vi "RemovePMUModule.vi"(8 "Error In":errorcluster[](array[cluster]), 11 "Bus in":refnum<class "Bus.lvclass">) -> (0 "Error Out":errorcluster[](array[cluster]), 3 "Bus out":refnum<class "Bus.lvclass">)   [LabVIEW 2014]
uses:
  Bus.lvclass
  <userlib>/NIST/NistModuleAdminLib/NistModuleAdmin/NistModuleAdmin.lvclass
  <userlib>/NIST/NISTErrorLib/NISTErrorLib.lvlib
  PmuImpairment/PmuImpairModule/PmuImpairModule.lvlib
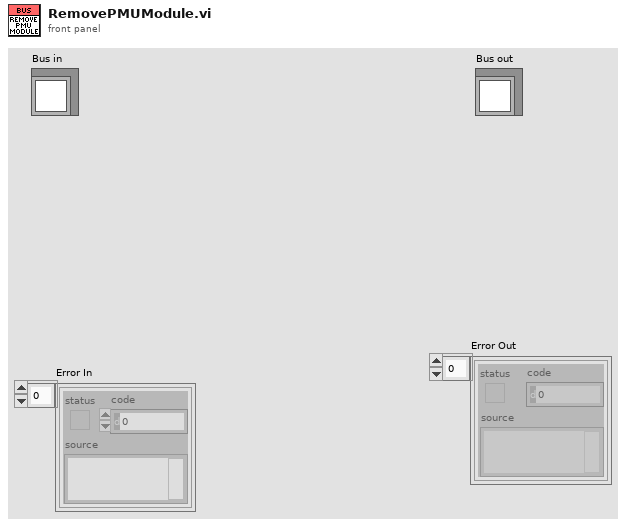
[diagram p1: front panel]
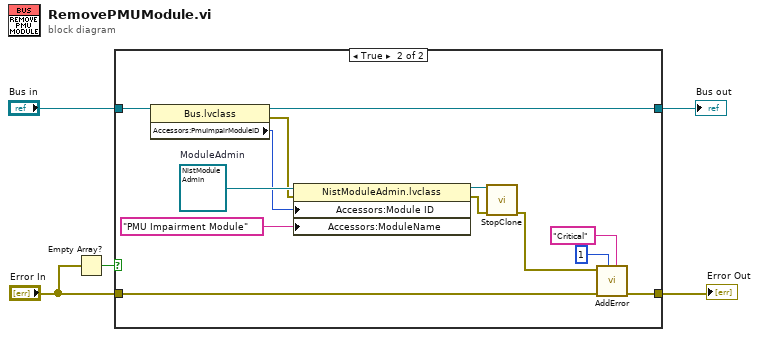
[diagram p0: block diagram]
diagram:
  n1 = Empty Array?(array="Error In") -> (empty?=w3:bool)
  n2 = case shown="True" w3 {
    tunnel: [w7 w8] -> w4
    tunnel: "Bus in" -> [w7 w20]
    tunnel: "Error In" -> [w6 w9]
    tunnel: [w6 w13] -> w1
    frame False {
    }
    frame True {
      w19 = refnum<class "NistModuleAdmin.lvclass"> refnum  # ModuleAdmin
      n3 = property class="Bus.lvclass"(reference=w20) -> (reference out=w8:refnum<class "Bus.lvclass">, error out=w14:errorcluster, "Accessors:PmuImpairModuleID"=w18:i32)  [unwired: 1 in]
      n4 = property class="NistModuleAdmin.lvclass"(reference=w19, error in=w14, "Accessors:Module ID"=w18, "Accessors:ModuleName"="PMU Impairment Module" ("ModuleName")) -> (reference out=w16:refnum<class "NistModuleAdmin.lvclass">, error out=w15:errorcluster)
      n5 = call "StopClone.vi"("error in (no error)"=w15, "ModuleAdmin"=w16) -> ("error out"=w10:errorcluster)  [unwired: 9 in]
      n6 = call <userlib>:"AddError.vi"("Severity"="Critical", "Priority"=u8 1, "ErrorArray"=w9, "error in (no error)"=w10) -> ("ErrorArray"=w13:errorcluster[])  [unwired: 6 in, 1 out]
    }
  }
  "Bus out" <- w4
  "Error Out" <- w1
